vi "VI Server_Cluster_GetVI ServerRefs.vi"(7 "Cluster.Label":string, 8 "error in":errorcluster, 11 "VI Server Cluster":T1) -> (0 "error out":errorcluster, 1 "Cluster_VI ServerRefs":T1={"Labels"=["Label", "Size", "Font", "Heght", "Width", "Ledding Denominator", "Ledding Nominator", "Label Number", "Microstep Resolution", "X", "Y", "Z", "Italic?", "Underlined?"], "Refs"=[], "VI Ref"=refnum}, 3 "VI Server Cluster.DUP":T1)   [LabVIEW 2020, in "VI Server Toolkit LV2013.lvlib"]
doc: "Retrieves VI Server Cluster value.\nUsed in the case multiple VI Server Clusters are being used - in the case of dynamically called VIs, for an example."
uses:
  VI Server Toolkit LV2013.lvlib
  VI Server_TypeDefs/VI Server_RefsCluster.ctl
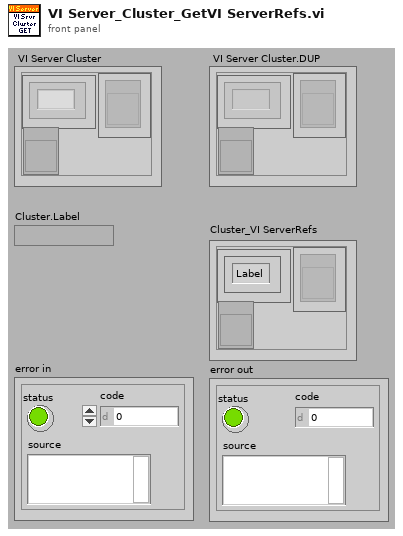
[diagram p1: front panel]
types:
  T1 = typedef "VI Server_RefsCluster.ctl" = cluster{"Labels":string[], "Refs":refnum<vi>[], "VI Ref":refnum<vi>}
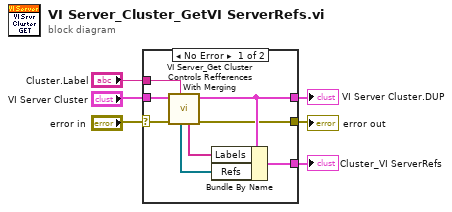
[diagram p0: block diagram]
diagram:
  n1 = case shown="No Error" "error in" {
    selector: "error in" -> [w10 w15]
    tunnel: "Cluster.Label" -> [w14 _]
    tunnel: [w13 _] -> w6
    tunnel: "VI Server Cluster" -> [w12 _]
    tunnel: [w11 w15] -> w4
    tunnel: [w9 _] -> w1
    frame No Error {
      n2 = call "VI Server_Get Cluster Controls Refferences With Merging.vi"("Cluster Label"=w14, "error in"=w10, "VI Server Cluster"=w12) -> ("error out"=w11:errorcluster, "VI Server Cluster.DUP"=w13:T1, "Claster.ControlLabels"=w8:string[], "Claster.ControRefs"=w7:refnum<vi>[])  [unwired: 5 out]
      n3 = Bundle By Name(cluster=w13, "Labels"=w8, "Refs"=w7) -> (w9:T1)
    }
    frame Error {
    }
  }
  "VI Server Cluster.DUP" <- w6
  "error out" <- w4
  "Cluster_VI ServerRefs" <- w1
